vi "Clear.vi"(3 "WavBuf":refnum<class "WavBuf.lvclass">) -> (1 "WavBuf Out":refnum<class "WavBuf.lvclass">)   [LabVIEW 2020, in "WavBuf.lvclass"]
uses:
  WavBuf.lvclass
  WavBuf.lvclass/WavBuf.ctl
  Universal Controls/Read Write Button.ctl
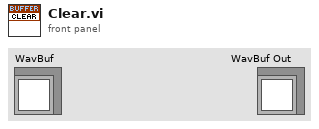
[diagram p1: front panel]
types:
  T1 = typedef "Read Write Button.ctl" = bool
  T2 = typedef "Ref_DVR_Buffer.ctl" = refnum<data-value>
  T3 = typedef "Waveform_Data.ctl" = waveform(dbl)
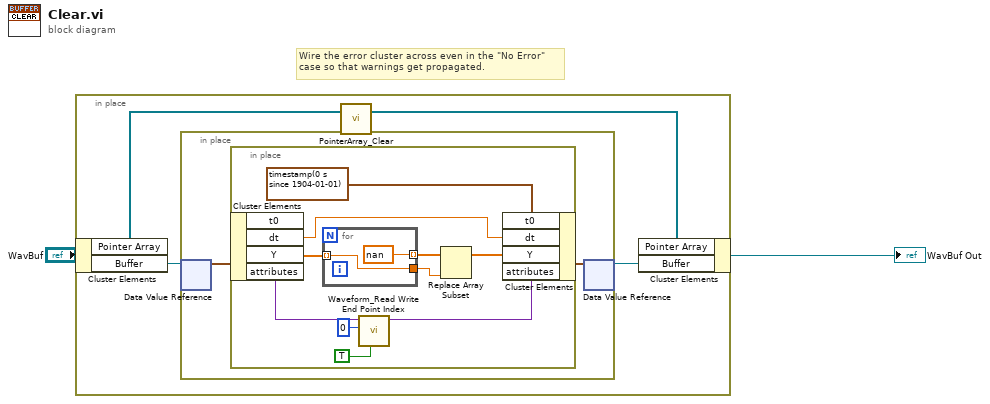
[diagram p0: block diagram]
diagram:
  # "Wire the error cluster across even in the \"No Error\"\ncase so that warnings get propagated."
  n1 = in-place {
    n2 = in-place-cluster #1("WavBuf") -> ("Pointer Array"=w6:refnum<class "_Pointer.lvclass">[], "Buffer"=w4:T2)
    n3 = in-place {
      n4 = in-place-dvr #2(w4) -> (w8:T3)  [unwired: 1 out]
      n5 = in-place {
        n6 = in-place-cluster #3(w8) -> ("dt"=w11:dbl, "Y"=w18:dbl[], "attributes"=w16:variant)  [unwired: 1 out]
        n7 = for {
          tunnel: w18 -> [w19] mode=indexing
          tunnel: [nan] -> w17 mode=indexing
          tunnel: [w19] -> w9
        }
        n8 = call "Waveform_Read Write End Point Index.vi"("Read(f)\nWrite(t)"=T1 TRUE ("Read(f)\nWrite(t)"), "End Point"=0, "Waveform Attributes"=w16) -> ("Waveform Attributes Out"=w15:variant)  [unwired: 5 in, 3 out]
        n9 = Replace Array Subset(array=w17, new element=w9) -> (w10:dbl[])  [unwired: 1 in]
        n10 = in-place-cluster #3("t0"=timestamp(0 s since 1904-01-01), "dt"=w11, "Y"=w10, "attributes"=w15) -> (w7:T3)
      }
      n11 = in-place-dvr #2(w7) -> (w3:T2)  [unwired: 1 out]
    }
    n12 = call "PointerArray_Clear.vi"("Pointer Array"=w6) -> ("Pointer Array Out"=w5:refnum<class "_Pointer.lvclass">[])  [unwired: 2 in]
    n13 = in-place-cluster #1("Pointer Array"=w5, "Buffer"=w3) -> (→"WavBuf Out":refnum<class "WavBuf.lvclass">)
  }
